vi "Create.vi"   [LabVIEW 2018, in "Toolkit.lvlib" / "File Info.lvclass"]
doc: "Creates a new File Info object and allocates memory within the libssh2lv shared library for a File Info struct."
uses:
  File Info.lvclass
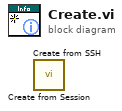
[diagram p0: block diagram]
diagram:
  n1 = call "Create from Session.vi"() -> ()  [unwired: 9 in, 3 out]
  n2 = call "Create from SSH.vi"() -> ()  [unwired: 10 in, 2 out]
